vi "Pomiar.vi"(0 "Voltage":dbl, 1 "Resistance":dbl, 2 "error in (no error)":errorcluster) -> (3 "Voltage output":dbl, 4 "Current output":dbl, 5 "error out":errorcluster)   [LabVIEW 2020]
doc: "Sub VI for single measurment of voltage and current.\nInputs:\n- Voltage set for power suply,\n- Resistance,\nOutputs:\n- Circut current\n- Diode voltage"
uses:
  VirtualLab.lvlibp/VISASimulator/VISALib.lvlib
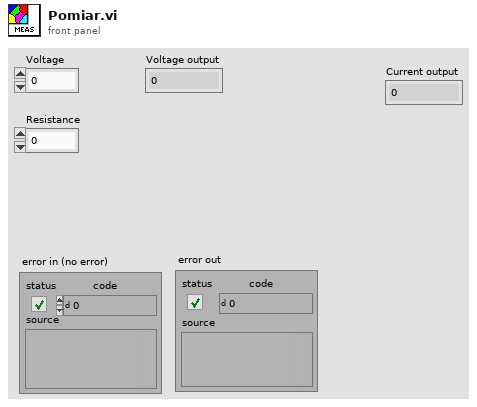
[diagram p1: front panel]
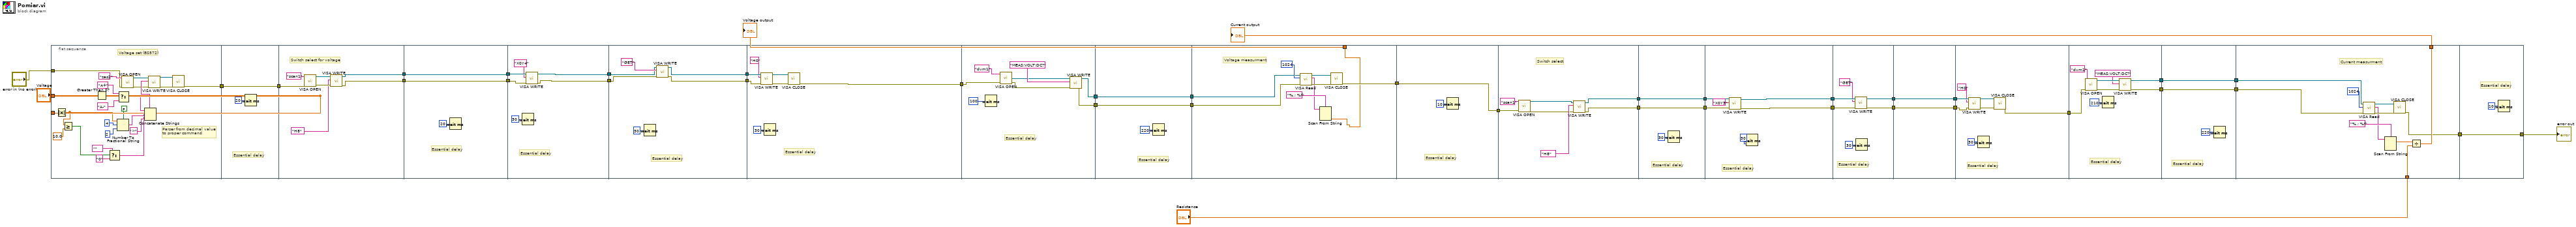
[diagram p0: block diagram]
diagram:
  n1 = flat-sequence {
    tunnel: "Voltage" -> [w50]
    tunnel: "Voltage" -> [w57]
    tunnel: "error in (no error)" -> [w41]
    tunnel: [w40] -> w33
    tunnel: [w65] -> w34
    tunnel: w33 -> [w65]
    tunnel: w34 -> [w69]
    tunnel: [w68] -> w20
    tunnel: [w67] -> w19
    tunnel: [w76] -> w5
    tunnel: w20 -> [w76]
    tunnel: [w75] -> w4
    tunnel: w19 -> [w75]
    tunnel: [w82] -> w3
    tunnel: [w81] -> w2
    tunnel: w4 -> [w80]
    tunnel: w5 -> [w79]
    tunnel: [w88] -> w17
    tunnel: [w87] -> w16
    tunnel: w2 -> [w85]
    tunnel: w3 -> [w84]
    tunnel: [w95] -> w18
    tunnel: w16 -> [w91]
    tunnel: w17 -> [w92]
    tunnel: w18 -> [w102]
    tunnel: [w99] -> w28
    tunnel: [w98] -> w26
    tunnel: w28 -> [w106]
    tunnel: [w106] -> w27
    tunnel: w26 -> [w105]
    tunnel: [w105] -> w25
    tunnel: [w107] -> w38
    tunnel: [w111] -> w31
    tunnel: w27 -> [w110]
    tunnel: w25 -> [w109]
    tunnel: [w116] -> w32
    tunnel: w31 -> [w116]
    tunnel: w32 -> [w122]
    tunnel: [w119] -> w14
    tunnel: [w118] -> w12
    tunnel: [w127] -> w15
    tunnel: w14 -> [w127]
    tunnel: [w126] -> w13
    tunnel: w12 -> [w126]
    tunnel: [w133] -> w11
    tunnel: [w132] -> w10
    tunnel: w13 -> [w131]
    tunnel: w15 -> [w130]
    tunnel: w11 -> [w136]
    tunnel: w10 -> [w139]
    tunnel: [w138] -> w9
    tunnel: [w137] -> w7
    tunnel: w9 -> [w141]
    tunnel: [w141] -> w8
    tunnel: w7 -> [w140]
    tunnel: [w140] -> w6
    tunnel: [w148] -> w1
    tunnel: w6 -> [w145]
    tunnel: w8 -> [w144]
    tunnel: w1 -> [w155]
    tunnel: [w150] -> w24
    tunnel: [w149] -> w22
    tunnel: w24 -> [w159]
    tunnel: [w159] -> w23
    tunnel: w22 -> [w158]
    tunnel: [w158] -> w21
    tunnel: "Resistance" -> [w166]
    tunnel: [w165] -> w36
    tunnel: [w164] -> w29
    tunnel: w23 -> [w161]
    tunnel: w21 -> [w160]
    tunnel: [w171] -> w30
    tunnel: w29 -> [w171]
    frame #0 {
      # "Parser from decimal value \nto proper command"
      # "Voltage set (BS572)"
      n2 = Absolute Value(x=w50) -> (abs(x)=w48:dbl)
      n3 = Greater Or Equal?(x=w48, y=10.0) -> (x >= y?=w51:bool)
      n4 = Greater Than 0?(x=w57) -> (x > 0?=w59:bool)
      n5 = Select(t="" ("string"), s=w51, f="0") -> (s? t:f=w44:string)
      n6 = Number To Fractional String(use system decimal point (T)=FALSE, number=w48, width (-)=i16 4, precision (6)=i16 2) -> (F-format string=w45:string)
      n7 = Select(t="A+" ("string"), s=w59, f="A-" ("string")) -> (s? t:f=w58:string)
      n8 = call "VISA OPEN.vi"("error in (no error)"=w41, "VISA resource name"="zas2") -> ("error out"=w55:errorcluster, "VISA resource name out"=w64:refnum<visa-resource-name>)  [unwired: 8 in]
      n9 = Concatenate Strings(w58, w44, w45, ">" ("string")) -> (w56:string)
      n10 = call "VISA WRITE.vi"("error in (no error)"=w55, "write buffer"=w56, "VISA resource name"=w64) -> ("error out"=w54:errorcluster, "VISA resource name out"=w63:refnum<visa-resource-name>)  [unwired: 6 in, 1 out]
      n11 = call "VISA CLOSE.vi"("error in (no error)"=w54, "VISA resource name"=w63) -> ("error out"=w40:errorcluster)  [unwired: 9 in]
    }
    frame #1 {
      # "Essential delay"
      n12 = Wait (ms)(milliseconds to wait=u32 20) -> ()  [unwired: 1 out]
    }
    frame #2 {
      # "Switch select for voltage"
      n13 = call "VISA OPEN.vi"("error in (no error)"=w69, "VISA resource name"="scan1") -> ("error out"=w72:errorcluster, "VISA resource name out"=w73:refnum<visa-resource-name>)  [unwired: 8 in]
      n14 = call "VISA WRITE.vi"("error in (no error)"=w72, "write buffer"="H8" ("string"), "VISA resource name"=w73) -> ("error out"=w68:errorcluster, "VISA resource name out"=w67:refnum<visa-resource-name>)  [unwired: 6 in, 1 out]
    }
    frame #3 {
      # "Essential delay"
      n15 = Wait (ms)(milliseconds to wait=u32 20) -> ()  [unwired: 1 out]
    }
    frame #4 {
      # "Essential delay"
      n16 = Wait (ms)(milliseconds to wait=u32 30) -> ()  [unwired: 1 out]
      n17 = call "VISA WRITE.vi"("error in (no error)"=w79, "write buffer"="X0Y4", "VISA resource name"=w80) -> ("error out"=w82:errorcluster, "VISA resource name out"=w81:refnum<visa-resource-name>)  [unwired: 6 in, 1 out]
    }
    frame #5 {
      # "Essential delay"
      n18 = Wait (ms)(milliseconds to wait=u32 30) -> ()  [unwired: 1 out]
      n19 = call "VISA WRITE.vi"("error in (no error)"=w84, "write buffer"="GET", "VISA resource name"=w85) -> ("error out"=w88:errorcluster, "VISA resource name out"=w87:refnum<visa-resource-name>)  [unwired: 6 in, 1 out]
    }
    frame #6 {
      # "Essential delay"
      n20 = call "VISA WRITE.vi"("error in (no error)"=w92, "write buffer"="H0", "VISA resource name"=w91) -> ("error out"=w93:errorcluster, "VISA resource name out"=w94:refnum<visa-resource-name>)  [unwired: 6 in, 1 out]
      n21 = Wait (ms)(milliseconds to wait=u32 30) -> ()  [unwired: 1 out]
      n22 = call "VISA CLOSE.vi"("error in (no error)"=w93, "VISA resource name"=w94) -> ("error out"=w95:errorcluster)  [unwired: 9 in]
    }
    frame #7 {
      # "Essential delay"
      n23 = Wait (ms)(milliseconds to wait=u32 100 ("millisecond timer value")) -> ()  [unwired: 1 out]
      n24 = call "VISA OPEN.vi"("error in (no error)"=w102, "VISA resource name"="dvm1") -> ("error out"=w101:errorcluster, "VISA resource name out"=w96:refnum<visa-resource-name>)  [unwired: 8 in]
      n25 = call "VISA WRITE.vi"("error in (no error)"=w101, "write buffer"="MEAS:VOLT:DC?", "VISA resource name"=w96) -> ("error out"=w99:errorcluster, "VISA resource name out"=w98:refnum<visa-resource-name>)  [unwired: 6 in, 1 out]
    }
    frame #8 {
      # "Essential delay"
      n26 = Wait (ms)(milliseconds to wait=u32 220) -> ()  [unwired: 1 out]
    }
    frame #9 {
      # "Voltage measurment"
      n27 = call "VISA Read.vi"("error in (no error)"=w110, "byte count"=u32 1024, "VISA resource name"=w109) -> ("error out"=w114:errorcluster, "read buffer"=w108:string, "VISA resource name out"=w115:refnum<visa-resource-name>)  [unwired: 5 in, 1 out]
      n28 = Scan From String(format string="%.; %f", input string=w108) -> (output 1=w107:dbl)  [unwired: 3 in, 3 out]
      n29 = call "VISA CLOSE.vi"("error in (no error)"=w114, "VISA resource name"=w115) -> ("error out"=w111:errorcluster)  [unwired: 9 in]
    }
    frame #10 {
      # "Essential delay"
      n30 = Wait (ms)(milliseconds to wait=u32 10) -> ()  [unwired: 1 out]
    }
    frame #11 {
      # "Switch select"
      n31 = call "VISA OPEN.vi"("error in (no error)"=w122, "VISA resource name"="scan1") -> ("error out"=w120:errorcluster, "VISA resource name out"=w121:refnum<visa-resource-name>)  [unwired: 8 in]
      n32 = call "VISA WRITE.vi"("error in (no error)"=w120, "write buffer"="H8" ("string"), "VISA resource name"=w121) -> ("error out"=w119:errorcluster, "VISA resource name out"=w118:refnum<visa-resource-name>)  [unwired: 6 in, 1 out]
    }
    frame #12 {
      # "Essential delay"
      n33 = Wait (ms)(milliseconds to wait=u32 30) -> ()  [unwired: 1 out]
    }
    frame #13 {
      # "Essential delay"
      n34 = call "VISA WRITE.vi"("error in (no error)"=w130, "write buffer"="X0Y3", "VISA resource name"=w131) -> ("error out"=w133:errorcluster, "VISA resource name out"=w132:refnum<visa-resource-name>)  [unwired: 6 in, 1 out]
      n35 = Wait (ms)(milliseconds to wait=u32 30) -> ()  [unwired: 1 out]
    }
    frame #14 {
      # "Essential delay"
      n36 = call "VISA WRITE.vi"("error in (no error)"=w136, "write buffer"="GET", "VISA resource name"=w139) -> ("error out"=w137:errorcluster, "VISA resource name out"=w138:refnum<visa-resource-name>)  [unwired: 6 in, 1 out]
      n37 = Wait (ms)(milliseconds to wait=u32 30) -> ()  [unwired: 1 out]
    }
    frame #15 {
    }
    frame #16 {
      # "Essential delay"
      n38 = call "VISA WRITE.vi"("error in (no error)"=w145, "write buffer"="H0", "VISA resource name"=w144) -> ("error out"=w146:errorcluster, "VISA resource name out"=w147:refnum<visa-resource-name>)  [unwired: 6 in, 1 out]
      n39 = Wait (ms)(milliseconds to wait=u32 30) -> ()  [unwired: 1 out]
      n40 = call "VISA CLOSE.vi"("error in (no error)"=w146, "VISA resource name"=w147) -> ("error out"=w148:errorcluster)  [unwired: 9 in]
    }
    frame #17 {
      # "Essential delay"
      n41 = call "VISA OPEN.vi"("error in (no error)"=w155, "VISA resource name"="dvm1") -> ("error out"=w154:errorcluster, "VISA resource name out"=w153:refnum<visa-resource-name>)  [unwired: 8 in]
      n42 = Wait (ms)(milliseconds to wait=u32 210) -> ()  [unwired: 1 out]
      n43 = call "VISA WRITE.vi"("error in (no error)"=w154, "write buffer"="MEAS:VOLT:DC?", "VISA resource name"=w153) -> ("error out"=w150:errorcluster, "VISA resource name out"=w149:refnum<visa-resource-name>)  [unwired: 6 in, 1 out]
    }
    frame #18 {
      # "Essential delay"
      n44 = Wait (ms)(milliseconds to wait=u32 220) -> ()  [unwired: 1 out]
    }
    frame #19 {
      # "Current measurment"
      n45 = call "VISA Read.vi"("error in (no error)"=w161, "byte count"=u32 1024, "VISA resource name"=w160) -> ("error out"=w169:errorcluster, "read buffer"=w162:string, "VISA resource name out"=w170:refnum<visa-resource-name>)  [unwired: 5 in, 1 out]
      n46 = Scan From String(format string="%.; %f", input string=w162) -> (output 1=w163:dbl)  [unwired: 3 in, 3 out]
      n47 = call "VISA CLOSE.vi"("error in (no error)"=w169, "VISA resource name"=w170) -> ("error out"=w164:errorcluster)  [unwired: 9 in]
      n48 = Divide(x=w163, y=w166) -> (x/y=w165:dbl)
    }
    frame #20 {
      # "Essential delay"
      n49 = Wait (ms)(milliseconds to wait=u32 10) -> ()  [unwired: 1 out]
    }
  }
  "Voltage output" <- w38
  "error out" <- w30
  "Current output" <- w36
